vi "GenerateName.vi"(9 "Rules":string[][](array[string]), 10 "Designator":string, 11 "Footprint":string) -> (3 "Name":string)   [LabVIEW 2015, in "ReportList.lvclass"]
uses:
  ReportList.lvclass
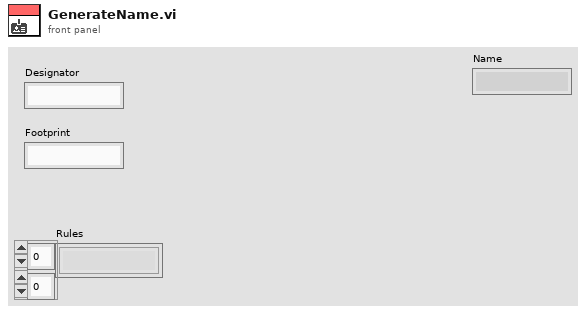
[diagram p1: front panel]
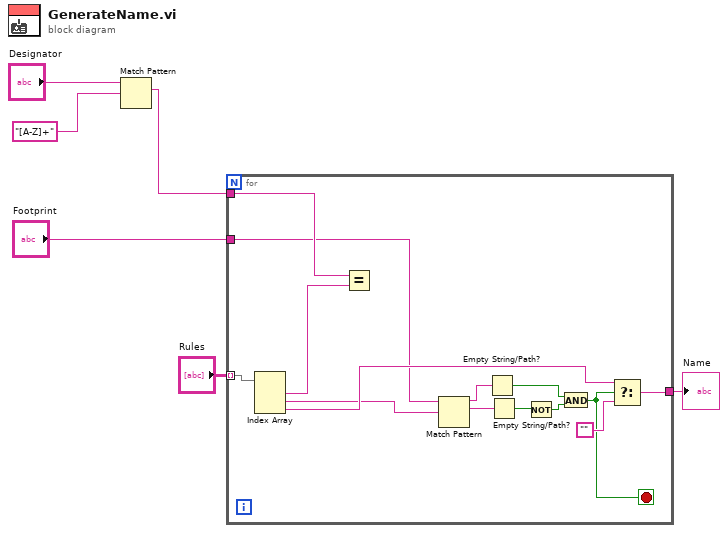
[diagram p0: block diagram]
diagram:
  n1 = Match Pattern(string="Designator", regular expression="[A-Z]+") -> (match substring=w4:string)  [unwired: 1 in, 3 out]
  n2 = for {
    tunnel: "Rules" -> [w19] mode=indexing
    tunnel: w4 -> [w20]
    tunnel: "Footprint" -> [w7]
    tunnel: [w10] -> w2
    stop <- w9 stop-if-true
    n3 = Index Array(array=w19) -> (element #1=w18:string, element #2=w8:string, element #3=w12:string)  [unwired: 3 in]
    n4 = Equal?(x=w20, y=w18) -> ()  [unwired: 1 out]
    n5 = Match Pattern(string=w7, regular expression=w8) -> (before substring=w16:string, match substring=w17:string)  [unwired: 1 in, 2 out]
    n6 = Empty String/Path?(string/path=w16) -> (empty?=w13:bool)
    n7 = Empty String/Path?(string/path=w17) -> (empty?=w15:bool)
    n8 = Not(x=w15) -> (.not. x?=w14:bool)
    n9 = And(x=w13, y=w14) -> (x .and. y?=w9:bool)
    n10 = Select(t=w12, s=w9, f="") -> (s? t:f=w10:string)
  }
  "Name" <- w2
